vi "Start Controller.vi"(8 "error in (no error)":errorcluster, 10 "Window Handle":i32, 11 "Config File Path":path=path "MeasurementConfig.ini") -> (0 "error out":errorcluster, 2 "Path to config file":path, 3 "Controller Queue":refnum<class "Message Enqueuer.lvclass">)   [LabVIEW 2026, in "Controller API.lvlib" / "Controller API.lvclass"]
doc: "This starts the controller that runs in the background to monitor running measurements and manage available resources. The path that is supplied to this method specifies the location of the configuration file. If it is not absolute, it will be appended to the disk location of this method. If the file does not exist at the specified location, it will be created using default settings."
uses:
  Controller API.lvclass
  Controller API.lvclass/Controller API.ctl
  framework/Msmt Configuration/Controller Configuration.lvclass
  framework/Controller/Controller.lvclass
  configuration/Configuration.lvclass
  <vilib>/ActorFramework/Actor/Actor.lvclass
  <vilib>/ActorFramework/Message Enqueuer/Message Enqueuer.lvclass
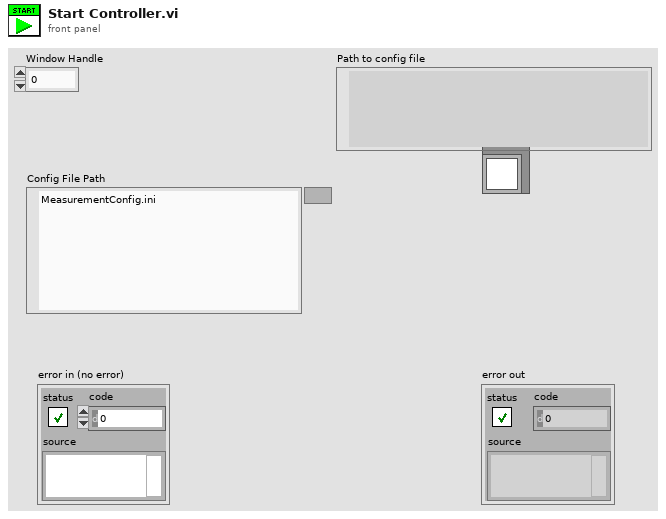
[diagram p1: front panel]
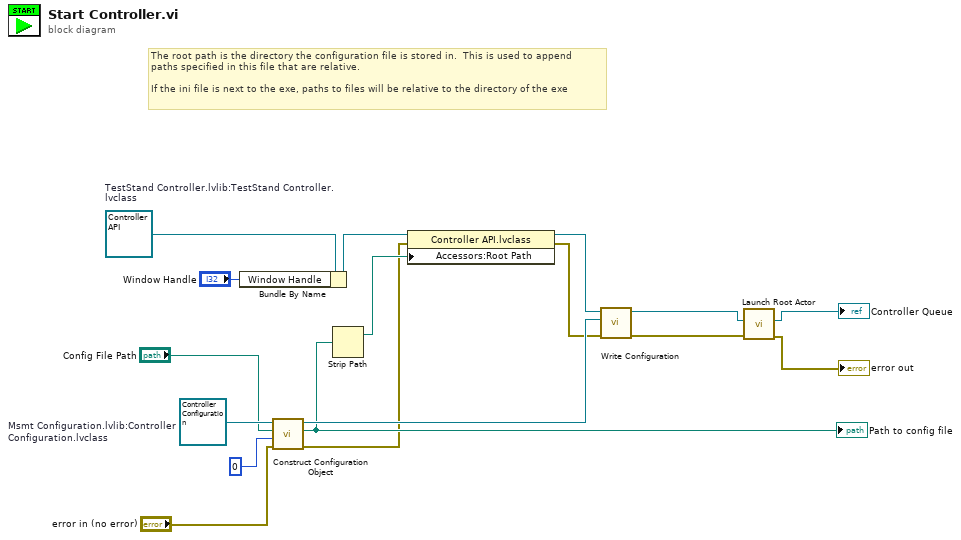
[diagram p0: block diagram]
diagram:
  w14 = refnum<class "Controller Configuration.lvclass"> refnum  # Msmt Configuration.lvlib:Controller Configuration.lvclass
  w12 = refnum<class "Controller API.lvclass"> refnum  # TestStand Controller.lvlib:TestStand Controller.lvclass
  # "The root path is the directory the configuration file is stored in.  This is used to append\npaths specified in this file that are relative.\n\nIf the ini file is next to the exe, paths to files will be relative to the directory of the exe"
  n1 = Bundle By Name(cluster=w12, "Window Handle"="Window Handle") -> (w11:refnum<class "Controller API.lvclass">)
  n2 = call "Construct Configuration Object.vi"("error in (no error)"="error in (no error)", "Initial Category Selection"=0, "Configuration File Path"="Config File Path", "Configuration in"=w14) -> ("error out"=w5:errorcluster, "Path to config file"=w7:path, "Configuration out"=w17:refnum<class "Controller Configuration.lvclass">)  [unwired: 4 in, 1 out]
  "Path to config file" <- w7
  n3 = Strip Path(path=w7) -> (stripped path=w13:path)  [unwired: 1 out]
  n4 = property class="Controller API.lvclass"(reference=w11, error in=w5, "Accessors:Root Path"=w13) -> (reference out=w16:refnum<class "Controller API.lvclass">, error out=w9:errorcluster)
  n5 = call "Write Configuration.vi"("error in (no error)"=w9, "Configuration.lvlib:Configuration.lvclass"=w17, "Controller in"=w16) -> ("error out"=w2:errorcluster, "Controller out"=w3:refnum<class "Controller API.lvclass">)  [unwired: 7 in]
  n6 = call <vilib>:"Launch Root Actor.vi"("error in (no error)"=w2, "Actor"=w3) -> ("error out"=→"error out":errorcluster, "Actor's Enqueuer"=→"Controller Queue":refnum<class "Message Enqueuer.lvclass">)  [unwired: 8 in]
